vi "FileHandlerQueue.vi"(7 "error in":errorcluster) -> (0 "error out":errorcluster, 3 "queue out":refnum<queue>)   [LabVIEW 2014]
uses:
  Controls/FHandlerClusterTypedef.ctl
  Controls/FHandlerEnumTypedef.ctl
panel:
  # "Obtain Master Queue Reference"
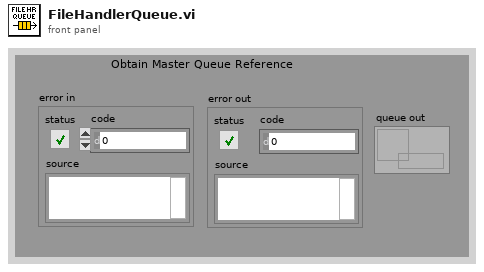
[diagram p1: front panel]
types:
  T1 = typedef "FHandlerClusterTypedef.ctl" = cluster{"File Variant":variant, "FileHandler Enum":T2}
  T2 = typedef "FHandlerEnumTypedef.ctl" = enum16{"InitLog", "CommentLog", "WriteExperimental", "WriteRGA", "WriteAccelerator", "WriteInstrument", "ClearLog", "ReadConfig", "WriteConfig", "ExitFH"}
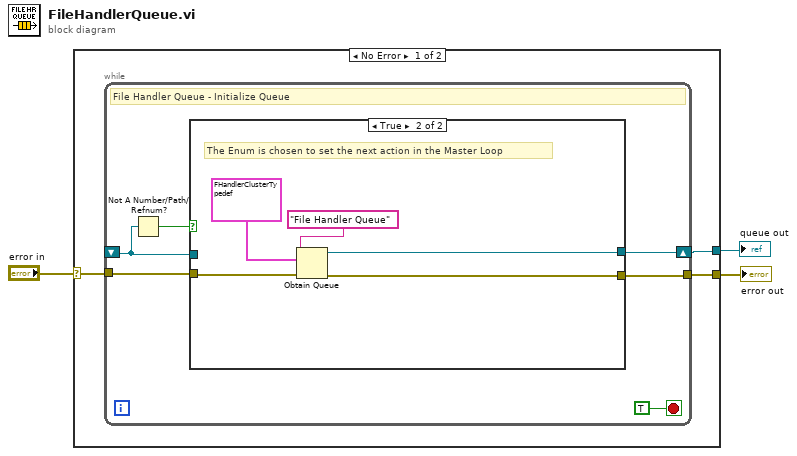
[diagram p0: block diagram]
diagram:
  n1 = case shown="No Error" "error in" {
    selector: "error in" -> [w4 w20]
    tunnel: [w6 w20] -> w3
    tunnel: [w5 _] -> w1
    frame No Error {
      n2 = while {
        shift-right: [w11] -> w5
        shift-left: _ -> [w8]
        tunnel: w4 -> [w10]
        tunnel: [w9] -> w6
        stop <- TRUE stop-if-true
        # "File Handler Queue - Initialize Queue"
        n3 = Not A Number/Path/Refnum?(number/path/refnum=w8) -> (NaN/Path/Refnum?=w7:bool)
        n4 = case shown="True" w7 {
          tunnel: [w14 w18] -> w11
          tunnel: w8 -> [w14 _]
          tunnel: w10 -> [w13 w19]
          tunnel: [w13 w17] -> w9
          frame False {
          }
          frame True {
            # "The Enum is chosen to set the next action in the Master Loop"
            n5 = Obtain Queue(name (unnamed)="File Handler Queue", element data type=T1 {"File Variant"=variant, "FileHandler Enum"=enum."InitLog"}, error in (no error)=w19) -> (queue out=w18:refnum<queue>, error out=w17:errorcluster)  [unwired: 2 in, 1 out]
          }
        }
      }
    }
    frame Error {
    }
  }
  "error out" <- w3
  "queue out" <- w1
